vi "BuildErrorLog.vi"(10 "Error Type":string, 11 "ROS":T1) -> (3 "error log path":path)   [LabVIEW 2012]
uses:
  SubVIs/_ROSDirection.ctl
  SubVIs/_ROSControl.ctl
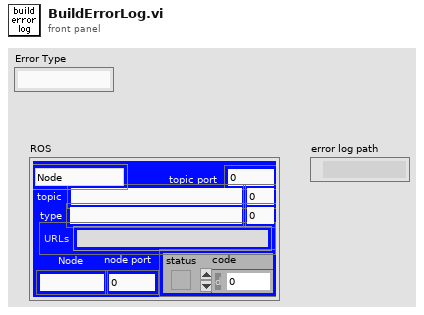
[diagram p1: front panel]
types:
  T1 = typedef "_ROSControl.ctl" = cluster{"topic port":u16, "Node":string, "topic":string, "type":string, "node port":u32, "error ":errorcluster, "Direction":T2, "APIs":string[], "Update (ms)":u16, "write queue":u16}
  T2 = typedef "_ROSDirection.ctl" = enum16{"Node", "Publisher", "Subscriber", "Service Client"}
  T3 = enum16{"open", "replace", "create", "open or create", "replace or create", "replace or create with confirmation"}
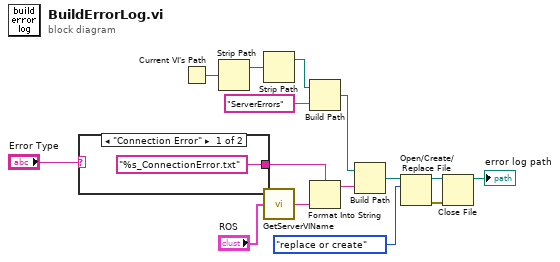
[diagram p0: block diagram]
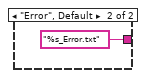
[diagram p2: hidden frame]
diagram:
  n1 = case shown="\"Connection Error\"" "Error Type" {
    tunnel: ["%s_ConnectionError.txt" ("format string") "%s_Error.txt" ("format string")] -> w14
    frame "Connection Error" {
    }
    frame "Error", Default {
    }
  }
  n2 = Current VI's Path() -> (path=w11:path)
  n3 = Strip Path(path=w11) -> (stripped path=w5:path)  [unwired: 1 out]
  n4 = Strip Path(path=w5) -> (stripped path=w4:path)  [unwired: 1 out]
  n5 = call "GetServerVIName.vi"("ROS"="ROS") -> ("vi name"=w13:string)
  n6 = Build Path(base path=w4, name or relative path="ServerErrors") -> (appended path=w3:path)
  n7 = Format Into String(format string=w14, w13) -> (resulting string=w15:string)  [unwired: 2 in, 1 out]
  n8 = Build Path(base path=w3, name or relative path=w15) -> (appended path=w8:path)
  n9 = Open/Create/Replace File(file path (use dialog)=w8, operation (0:open)=T3."replace or create") -> (refnum out=w9:refnum<file>, error out=w10:errorcluster)  [unwired: 4 in, 1 out]
  n10 = Close File(refnum=w9, error in=w10) -> (path=→"error log path":path)  [unwired: 1 out]
